vi "Write Position.vi"(8 "error in (no error)":errorcluster, 9 "Position":T1, 10 "Session In":refnum<class "Session.lvclass">, 11 "Grove I2C LCD I in":refnum<class "Grove I2C LCD.lvclass">) -> (0 "error out":errorcluster, 2 "Session Out":refnum<class "Session.lvclass">, 3 "Grove I2C LCD I out":refnum<class "Grove I2C LCD.lvclass">)   [LabVIEW 2020, in "CTI-Peripheral.lvlib" / "Grove I2C LCD.lvclass"]
uses:
  Grove I2C LCD.lvclass
  Character LCD/Position.ctl
  CTI/Session/Session.lvclass
  Character LCD/Char LCD.lvclass
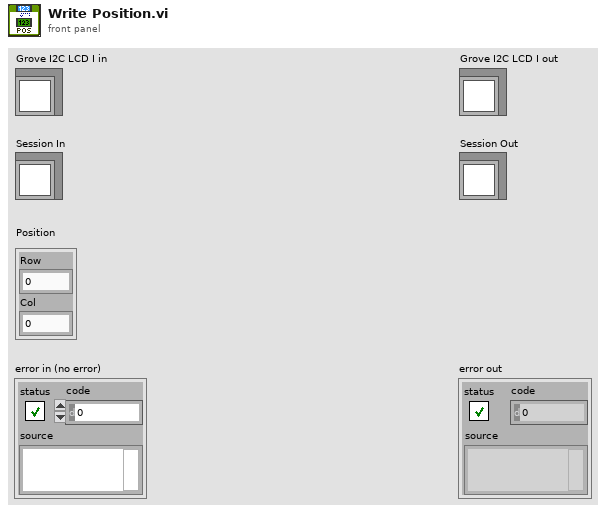
[diagram p1: front panel]
types:
  T1 = typedef "CTI-Peripheral.lvlib/Char LCD.lvclass/Position.ctl" = cluster{"Row":u8, "Col":u8}
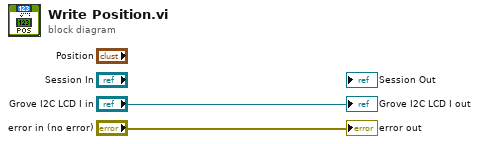
[diagram p0: block diagram]
diagram:
  "error out" <- "error in (no error)"
  "Grove I2C LCD I out" <- "Grove I2C LCD I in"
